vi "Pre-Dig Hook.vi"(8 "Error In":errorcluster) -> (0 "Error Out":errorcluster)   [LabVIEW 2018, in "Tests.lvlib" / "Toolkit.lvlib" / "Integration.lvlib"]
uses:
  Integration.lvlib
  Hooks/Pre-Dig/Pre-Dig.vi
  src/Toolkit/Toolkit.lvlib
  <vilib>/addons/_JKI Toolkits/Caraya/classes/Test/Test.lvclass
  Tests.lvlib
  <vilib>/addons/_JKI Toolkits/Caraya/classes/Assert/Assert.lvclass
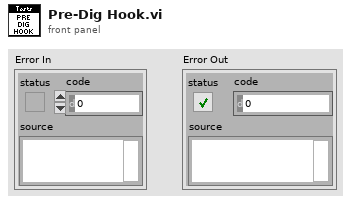
[diagram p1: front panel]
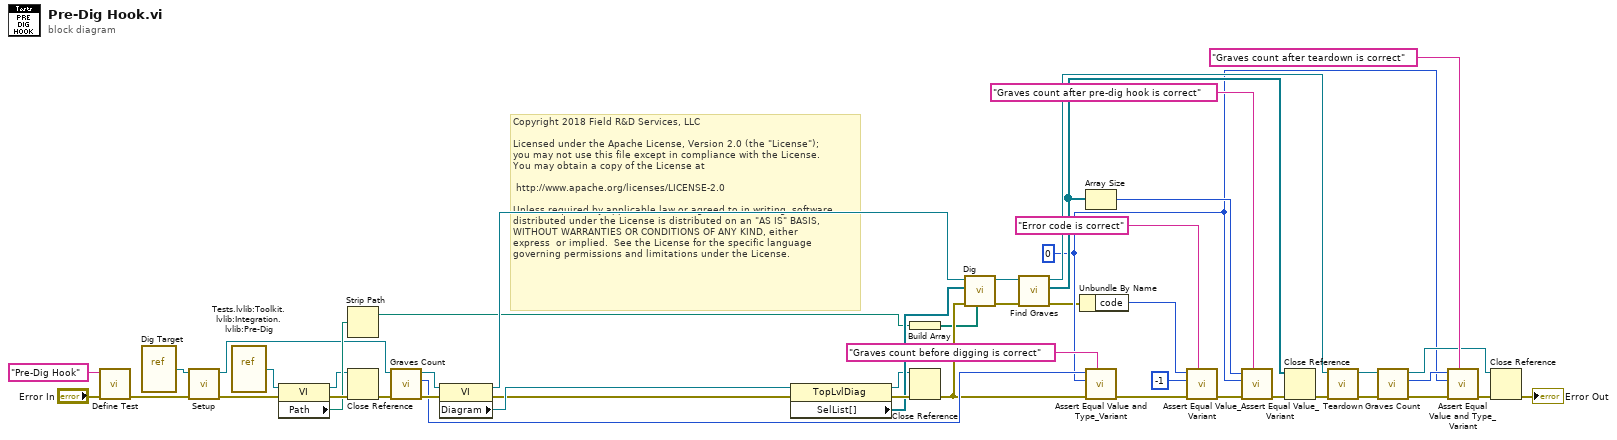
[diagram p0: block diagram]
diagram:
  w7 = 0 ("size(s)")
  # "Copyright 2018 Field R&D Services, LLC\n\nLicensed under the Apache License, Version 2.0 (the \"License\");\nyou may not use this file except in compliance with the License.\nYou may obtain a copy of the License at\n\n\thttp://www.apache.org/licenses/LICENSE-2.0\n\nUnless required by applicable law or agreed to in writing, software\ndistributed under the License is distributed on an \"AS IS\" BASIS,\nWITHOUT WARRANTIES OR CONDITIONS OF ANY KIND, either \nexpress  or implied.  See the License for the specific language \ngoverning permissions and limitations under the License."
  n1 = call <vilib>:"Define Test.vi"("error in (no error)"="Error In", "Label (VI Title)"="Pre-Dig Hook") -> ("error out"=w26:errorcluster)  [unwired: 9 in]
  n2 = vi-ref "Dig Target.vi"() -> (w44:refnum<vi>)
  n3 = call "Setup.vi"("Error In"=w26, "VI In"=w44) -> ("Error Out"=w13:errorcluster, "VI Out"=w2:refnum<vi>)  [unwired: 8 in]
  n4 = vi-ref "Tests.lvlib:Toolkit.lvlib:Integration.lvlib:Pre-Dig.vi"() -> (w1:refnum<vi>)
  n5 = property class="VI"(reference=w1, error in=w13) -> (reference out=w8:refnum<vi>, error out=w12:errorcluster, "Path"=w11:path)
  n6 = Strip Path(path=w11) -> (stripped path=w10:path)  [unwired: 1 out]
  n7 = Close Reference(reference=w8, error in (no error)=w12) -> (error out=w9:errorcluster)
  n8 = call "Graves Count.vi"("Error In"=w9, "Test Target In"=w2) -> ("Error Out"=w23:errorcluster, "Graves Count"=w22:i32, "Test Target Out"=w27:refnum<vi>)  [unwired: 7 in]
  n9 = property class="VI"(reference=w27, error in=w23) -> (reference out=w43:refnum<vi>, error out=w46:errorcluster, "Diagram"=w47:refnum<vi>)
  n10 = property class="TopLvlDiag"(reference=w47, error in=w46) -> (reference out=w36:refnum<vi>, error out=w45:errorcluster, "SelList[]"=w42:refnum<vi>[])
  n11 = Build Array(w10) -> (w3:path[])
  n12 = Close Reference(reference=w36, error in (no error)=w45) -> (error out=w19:errorcluster)
  n13 = call "Dig.vi"("Hooks Search Path"=w3, "Error In"=w19, "Selection List[]"=w42, "VI In"=w43) -> ("Error Out"=w41:errorcluster, "VI Out"=w28:refnum<vi>)  [unwired: 6 in]
  n14 = call "Find Graves.vi"("Error In"=w41, "VI In"=w28) -> ("Error Out"=w6:errorcluster, "Graves"=w30:refnum<vi>[], "VI Out"=w32:refnum<vi>)  [unwired: 7 in]
  n15 = Unbundle By Name(w6) -> ("code"=w5:i32)
  n16 = Array Size(array=w30) -> (size(s)=w35:i32)
  n17 = call <vilib>:"Assert Equal Value and Type_Variant.vi"("Label"="Graves count before digging is correct", "error in (no error)"=w19, "Y"=w7, "X"=w22) -> ("error out"=w25:errorcluster)  [unwired: 7 in]
  n18 = call <vilib>:"Assert Equal Value_Variant.vi"("Label"="Error code is correct", "error in (no error)"=w25, "Y"=-1 ("code"), "X"=w5) -> ("error out"=w38:errorcluster)  [unwired: 7 in]
  n19 = call <vilib>:"Assert Equal Value_Variant.vi"("Label"="Graves count after pre-dig hook is correct", "error in (no error)"=w38, "Y"=w7, "X"=w35) -> ("error out"=w33:errorcluster)  [unwired: 7 in]
  n20 = Close Reference(reference=w30, error in (no error)=w33) -> (error out=w29:errorcluster)
  n21 = call "Teardown.vi"("Error In"=w29, "VI In"=w32) -> ("Error Out"=w16:errorcluster, "VI Out"=w18:refnum<vi>)  [unwired: 8 in]
  n22 = call "Graves Count.vi"("Error In"=w16, "Test Target In"=w18) -> ("Error Out"=w15:errorcluster, "Graves Count"=w14:i32, "Test Target Out"=w17:refnum<vi>)  [unwired: 7 in]
  n23 = call <vilib>:"Assert Equal Value and Type_Variant.vi"("Label"="Graves count after teardown is correct", "error in (no error)"=w15, "Y"=w7, "X"=w14) -> ("error out"=w21:errorcluster)  [unwired: 7 in]
  n24 = Close Reference(reference=w17, error in (no error)=w21) -> (error out=→"Error Out":errorcluster)
